vi "Format_USNO_data.vi"(4 "Data IN":string[][](array[string])) -> (1 "Data OUT":string[][](array[string]))   [LabVIEW 2011]
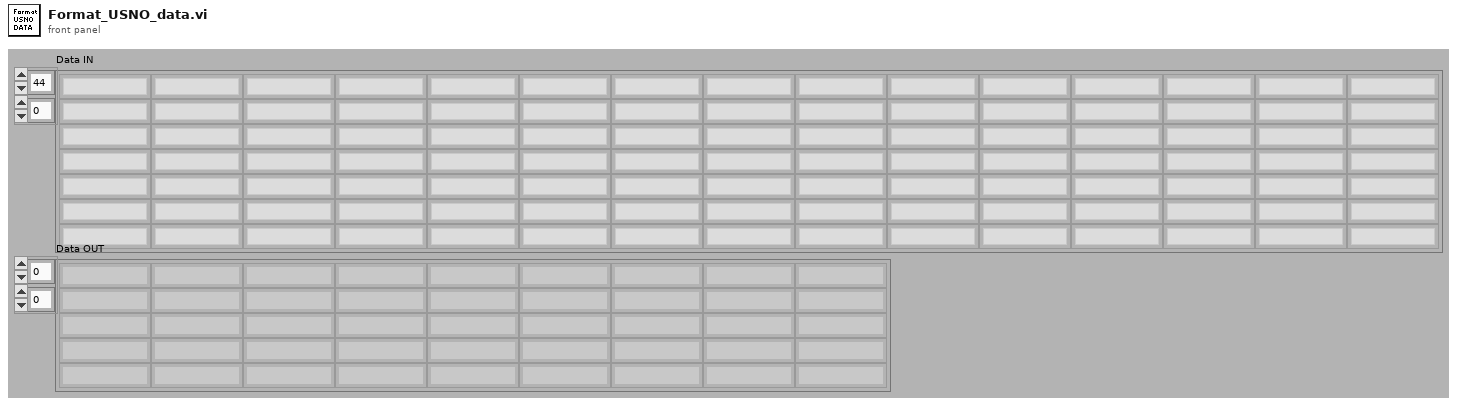
[diagram p1: front panel]
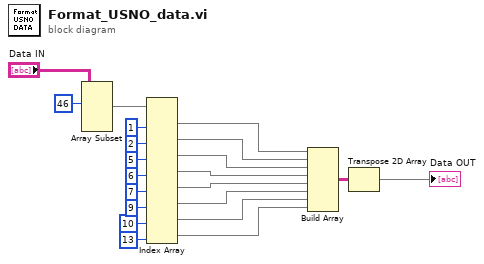
[diagram p0: block diagram]
diagram:
  n1 = Array Subset(array="Data IN", index (row)=46 ("index")) -> (w19:string[][])  [unwired: 3 in]
  n2 = Index Array(array=w19, index (col) #1=1 ("disabled index (col)"), index (col) #2=2 ("index (col)"), index (col) #3=5 ("index (col)"), index (col) #4=6 ("index (col)"), index (col) #5=7 ("index (col)"), index (col) #6=9 ("index (col)"), index (col) #7=10 ("index (col)"), index (col) #8=13 ("index (col)")) -> (element #1=w10:string[], element #2=w9:string[], element #3=w8:string[], element #4=w7:string[], element #5=w6:string[], element #6=w5:string[], element #7=w4:string[], element #8=w3:string[])  [unwired: 8 in]
  n3 = Build Array(w10, w9, w8, w7, w6, w5, w4, w3) -> (w2:string[][])
  n4 = Transpose 2D Array(2D array=w2) -> (transposed array=→"Data OUT":string[][])
